vi "Animaciones.vi"() -> ()   [LabVIEW 2017]
panel:
  out "Animaciones":cluster{"Trituradora":bool, " Caja":bool}
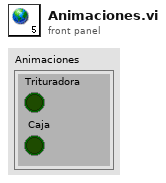
[diagram p1: front panel]
diagram:
